vi "a.vi"(10 "Numeric":dbl, 11 "reference 2":refnum<k7>) -> (3 "Boolean":bool)   [LabVIEW 2023]
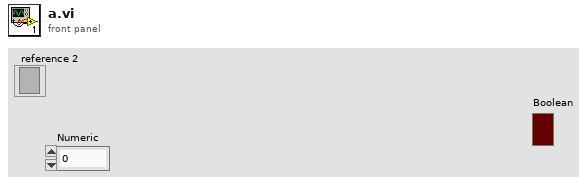
[diagram p1: front panel]
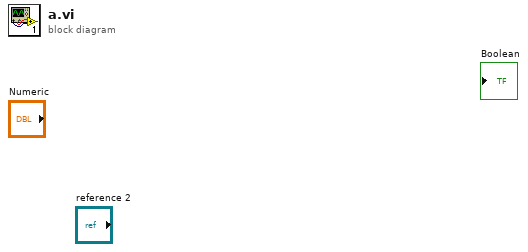
[diagram p0: block diagram]
diagram:
